vi "Get Node Outgoing Edges.vi"(8 "error in (no error)":errorcluster, 10 "Name":string, 11 "FSM in":refnum<class "FSM.Graph.lvclass">) -> (0 "error out":errorcluster, 2 "Edges":refnum<class "FSM.Edge.lvclass">[](array[class]), 3 "FSM out":refnum<class "FSM.Graph.lvclass">)   [LabVIEW 2015, in "FSM.Graph.lvclass"]
uses:
  FSM.Graph.lvclass
  FSM.Edge/FSM.Edge.lvclass
  FSM.Graph.lvclass/FSM.Graph.ctl
  FSM.Edge/FSM.Edge.lvclass/FSM.Edge.ctl
  FSM.Edge/Read SourceName.vi
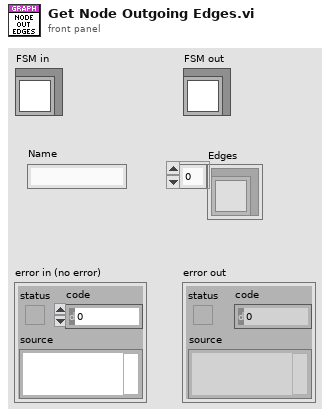
[diagram p1: front panel]
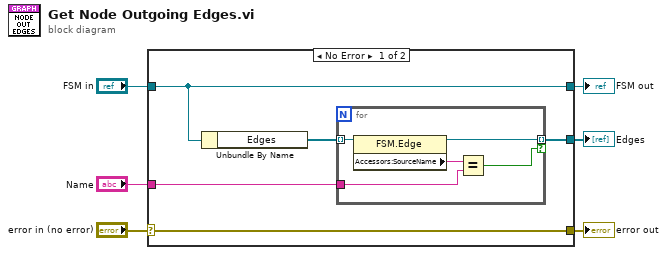
[diagram p0: block diagram]
diagram:
  n1 = case shown="No Error" "error in (no error)" {
    selector: "error in (no error)" -> [w11 w18]
    tunnel: [w11 w18] -> w5
    tunnel: [w10 w17] -> w3
    tunnel: "FSM in" -> [w10 w17]
    tunnel: "Name" -> [w8 _]
    tunnel: [w7 _] -> w1
    frame No Error {
      n2 = Unbundle By Name(w10) -> ("Edges"=w9:refnum<class "FSM.Edge.lvclass">[])
      n3 = for {
        tunnel: w9 -> [w16] mode=indexing
        tunnel: w8 -> [w14]
        tunnel: [w13] -> w7 mode=indexing if=w12
        n4 = property class="FSM.Edge"(reference=w16) -> (reference out=w13:refnum<class "FSM.Edge.lvclass">, "Accessors:SourceName"=w15:string)  [unwired: 1 in, 1 out]
        n5 = Equal?(x=w15, y=w14) -> (x = y?=w12:bool)
      }
    }
    frame Error {
    }
  }
  "error out" <- w5
  "FSM out" <- w3
  "Edges" <- w1
